vi "DecodeChannelSettings.vi"(0 "Highland T564 DDG in":refnum<class "Highland T564 DDG.lvclass">, 5 "Channel":string, 7 "PropertyLabel":string, 9 "ElementValue":string, 11 "error in (no error)":errorcluster) -> (4 "Highland T564 DDG out":refnum<class "Highland T564 DDG.lvclass">, 15 "error out":errorcluster)   [LabVIEW 2020, in "Highland T564 DDG.lvclass"]
uses:
  Highland T564 DDG.lvclass
  C:/GEECS/Developers Version/source/Device Drivers/shared/MetaDriver_v1/MetaDriver_v1.lvclass
  Choice83.ctl
  Choice84.ctl
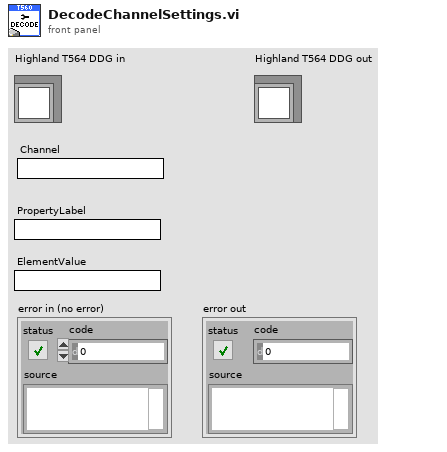
[diagram p1: front panel]
types:
  T1 = typedef "Choice83.ctl" = enum16{"Direct", "Inverted"}
  T2 = typedef "Choice84.ctl" = enum16{"Null", "A", "B", "C", "D", "Trigger"}
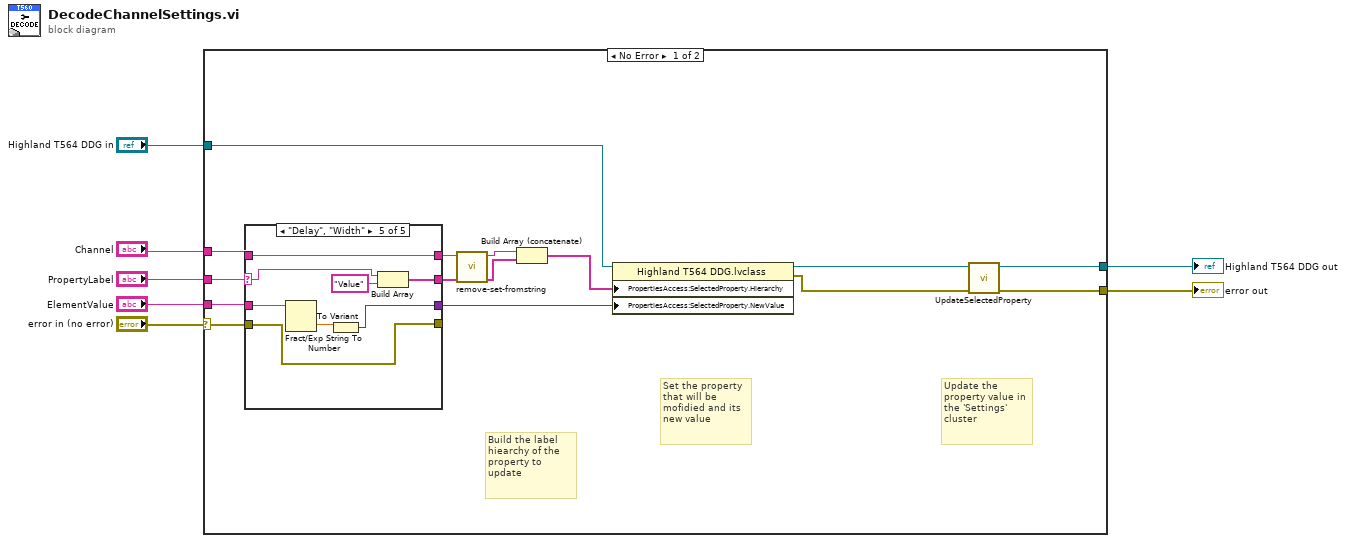
[diagram p0: block diagram]
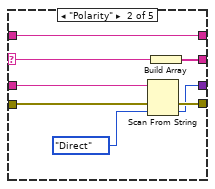
[diagram p3: hidden frame]
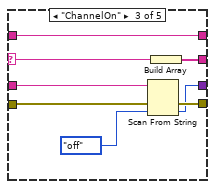
[diagram p4: hidden frame]
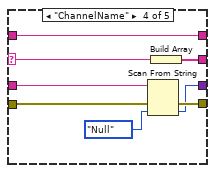
[diagram p5: hidden frame]
diagram:
  n1 = case shown="No Error" "error in (no error)" {
    selector: "error in (no error)" -> [w15 w55]
    tunnel: "PropertyLabel" -> [w21 _]
    tunnel: "ElementValue" -> [w20 _]
    tunnel: "Channel" -> [w17 _]
    tunnel: "Highland T564 DDG in" -> [w14 w54]
    tunnel: [w8 w54] -> w3
    tunnel: [w9 w55] -> w2
    frame No Error {
      # "Update the property value in the 'Settings' cluster"
      # "Set the property that will be mofidied and its new value"
      # "Build the label hiearchy of the property to update"
      n2 = case shown="\"Delay\", \"Width\"" w21 {
        selector: w21 -> [_ w27 w35 w44 w46]
        tunnel: w20 -> [_ w28 w36 w45 w51]
        tunnel: [_ w25 w33 w42 w48] -> _
        tunnel: [_ w26 w34 w43 w50] -> w18
        tunnel: w17 -> [_ w24 w32 w41 w49]
        tunnel: [_ w24 w32 w41 w49] -> w16
        tunnel: w15 -> [_ w23 w31 w40 w48]
        tunnel: [_ w22 w30 w38 w47] -> w12
        frame Default {
        }
        frame "Polarity" {
          n3 = Scan From String(input string=w28, error in=w23, default 1=Choice83."Direct" ("Polarity")) -> (error out=w25:errorcluster, output 1=w22:T1)  [unwired: 2 in, 2 out]
          n4 = Build Array(w27) -> (w26:string[])
        }
        frame "ChannelOn" {
          n5 = Scan From String(input string=w36, error in=w31, default 1=enum16{"off", "on"}."off" ("ON/OFF")) -> (error out=w33:errorcluster, output 1=w30:enum16{"off", "on"})  [unwired: 2 in, 2 out]
          n6 = Build Array(w35) -> (w34:string[])
        }
        frame "ChannelName" {
          n7 = Scan From String(input string=w45, error in=w40, default 1=Choice84."Null" ("ChannelName")) -> (error out=w42:errorcluster, output 1=w38:T2)  [unwired: 2 in, 2 out]
          n8 = Build Array(w44) -> (w43:string[])
        }
        frame "Delay", "Width" {
          n9 = Fract/Exp String To Number(string=w51) -> (number=w52:dbl)  [unwired: 3 in, 1 out]
          n10 = To Variant(anything=w52) -> (Variant=w47:variant)
          n11 = Build Array(w46, "Value" ("element")) -> (w50:string[])
        }
      }
      n12 = call "remove-set-fromstring.vi"("String"=w16) -> ("result string"=w19:string)  [unwired: 9 in, 1 out]
      n13 = Build Array (concatenate)(w19, w18) -> (w13:string[])
      n14 = property class="Highland T564 DDG.lvclass"(reference=w14, "PropertiesAccess:SelectedProperty.Hierarchy"=w13, "PropertiesAccess:SelectedProperty.NewValue"=w12) -> (reference out=w11:refnum<class "Highland T564 DDG.lvclass">, error out=w10:errorcluster)  [unwired: 1 in]
      n15 = call-dynamic "UpdateSelectedProperty.vi"("error in (no error)"=w10, "Highland T564 DDG in"=w11) -> ("error out"=w9:errorcluster, "Highland T564 DDG out"=w8:refnum<class "Highland T564 DDG.lvclass">)  [unwired: 8 in]
    }
    frame Error {
    }
  }
  "error out" <- w2
  "Highland T564 DDG out" <- w3
